vi "NumIntegrate_Rkdp_Func_B2.vi"(11 "Index":i32) -> (3 "RKDP_B2":dbl)   [LabVIEW 2019, in "Trajectory_Library.lvlib"]
doc: "Internal function used by Rkdp_Impl.vi\n\nInputs:\n - Index -- Index into B2 array (must be 0 - 6 )\n\nOutputs:\n - B2 -- Value looked up by index."
uses:
  Trajectory_Library.lvlib
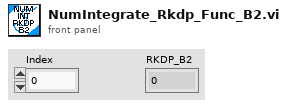
[diagram p1: front panel]
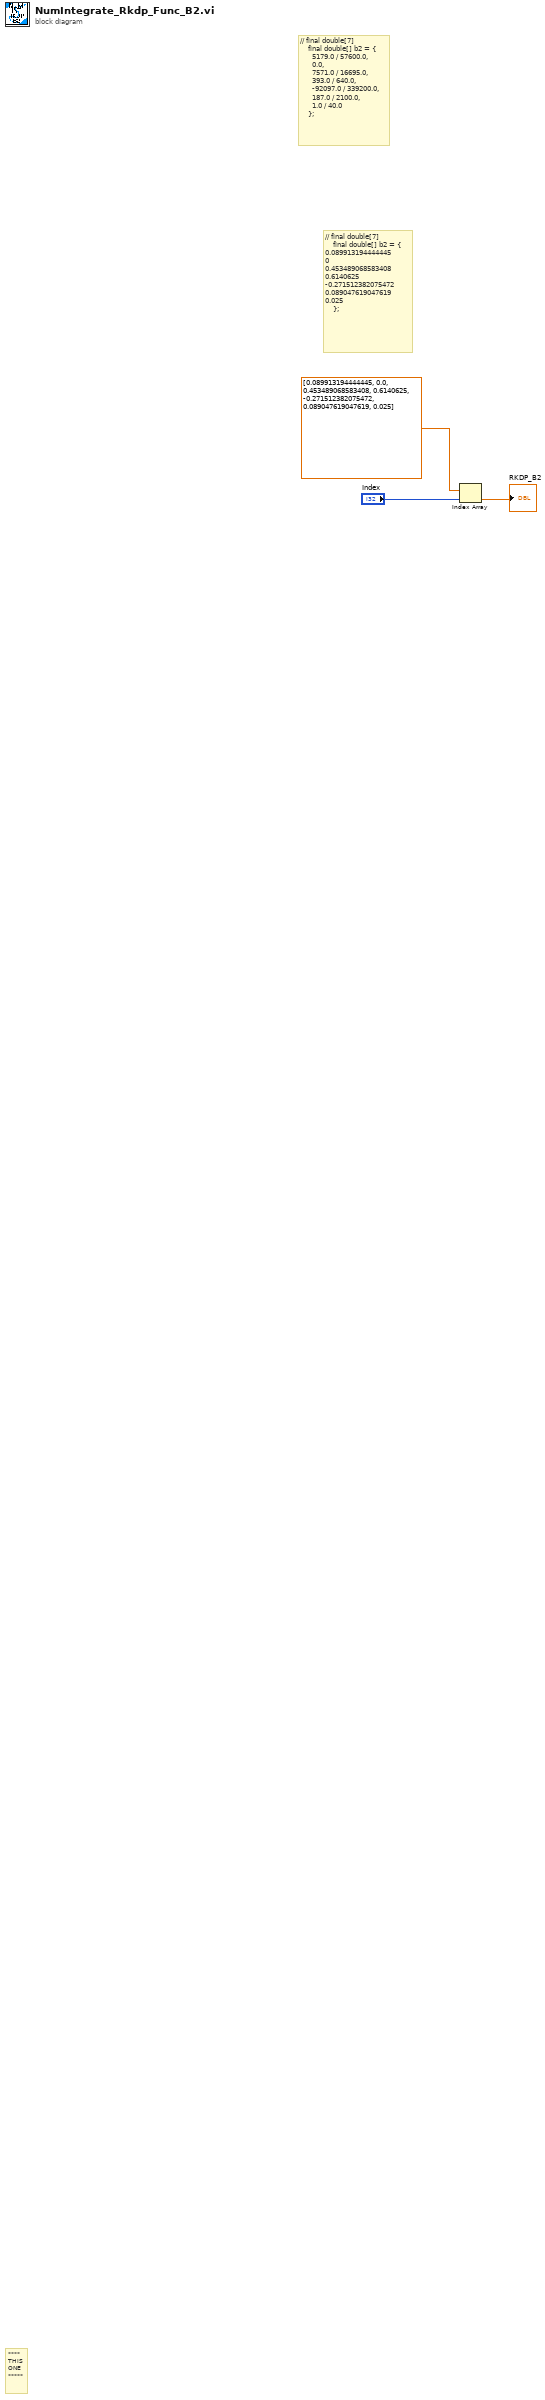
[diagram p0: block diagram]
diagram:
  # "// final double[7]\n    final double[] b2 = {\n0.089913194444445\n0\n0.453489068583408\n0.6140625\n-0.271512382075472\n0.089047619047619\n0.025\n    };"
  # "// final double[7]\n    final double[] b2 = {\n      5179.0 / 57600.0,\n      0.0,\n      7571.0 / 16695.0,\n      393.0 / 640.0,\n      -92097.0 / 339200.0,\n      187.0 / 2100.0,\n      1.0 / 40.0\n    };"
  # "****\nTHIS\nONE\n*****"
  n1 = Index Array(array=dbl[] [0.089913194444445, 0.0, 0.453489068583408, 0.6140625, -0.271512382075472, 0.089047619047619, 0.025], index="Index") -> (element=→"RKDP_B2":dbl)
